vi "SP Add Marker to Plots.vi"(5 "CH Control":T3={"Trace Orientation"=enum."Overlay", "Frequency"={"Change Frequency"=FALSE, "Start"=500.0, "Stop"=1500.0, "Units"=enum."MHz"}, "Markers"=[], "Traces"=[]} {"Traces"."Reference" format="%#.2g"; "Traces"."Display Data" items=["Data", "Memory", "Data/Memory"]; "Traces"."Format" items=["Log Mag", "Phase", "Expanded Phase", "Delay", "Smith", "Polar", "Lin Mag", "SWR", "Loss", "Real", "Imaginary"]; "Traces"."Scale" min=0.001 step=1.0 format="%#.2g"; "Traces"."Position" min=0.0 max=10.0; "Frequency"."Stop" format="%.3g"; "Frequency"."Start" format="%.3g"}, 7 "Plot References":refnum<vi>[](array[refnum]), 8 "error in (no error)":errorcluster, 9 "Marker":T1, 10 "Marker Table":refnum<vi>, 11 "Plot Ref":refnum<vi>) -> (0 "error out":errorcluster)   [LabVIEW 2011]
uses:
  TypeDefs/SP Display Plot Controls Cluster.ctl
  TypeDefs/SP Frequency Units.ctl
  TypeDefs/SP Marker Cluster.ctl
  TypeDefs/SP Marker Type.ctl
  TypeDefs/SP Display Trace Controls.ctl
  TypeDefs/SP Display Format.ctl
  TypeDefs/SP Display Data.ctl
panel:
  # "Div"
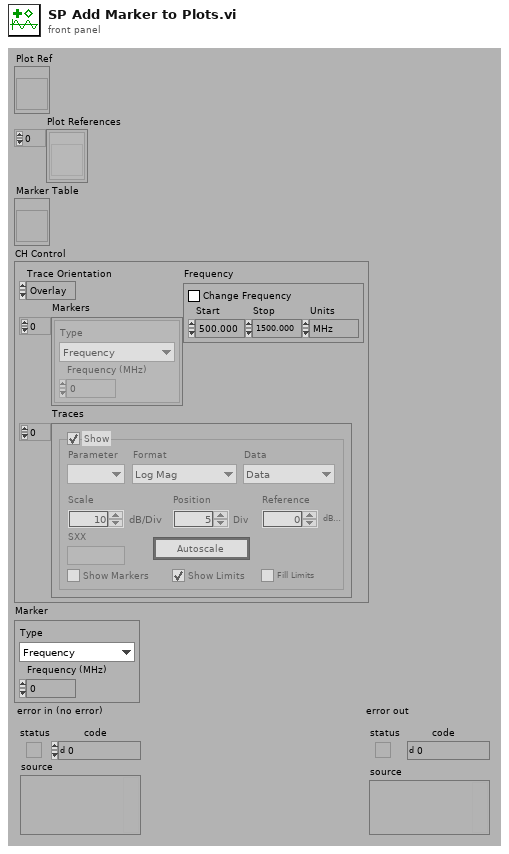
[diagram p1: front panel]
types:
  T1 = typedef "SP Marker Cluster.ctl" = cluster{"Type":T2, "Frequency (MHz)":dbl}
  T2 = typedef "SP Marker Type.ctl" = enum16{"Frequency", "Trace Maximum", "Trace Minimum", "Limit Maximum", "Limit Minimum"}
  T3 = typedef "SP Display Plot Controls Cluster.ctl" = cluster{"Trace Orientation":enum32{"Overlay", "Split"}, "Frequency":cluster{"Change Frequency":bool, "Start":dbl, "Stop":dbl, "Units":T4}, "Markers":T1[], "Traces":T5[]}
  T4 = typedef "SP Frequency Units.ctl" = enum16{"Hz", "kHz", "MHz", "GHz", "Points"}
  T5 = typedef "SP Display Trace Controls.ctl" = cluster{"Trace On":bool, "Measure":i32, "Format":T6, "Autoscale":bool, "Reference":dbl, "\nRefUnit":string, "Position":dbl, "Scale":dbl, "ScaleUnit":string, "LimitOn":bool, "LimitFill":bool, "Display Data":T7, "Show Markers":bool, "SXX":string}
  T6 = typedef "SP Display Format.ctl" = i32
  T7 = typedef "SP Display Data.ctl" = u16
  T8 = typedef "SP Channel Data.ctl" = cluster{"Graph Ref":refnum<vi>, "Data":cluster{"Data":cluster{"X":dbl[], "Y":dbl[]}, "Index":i32}, "ULimits":cluster{"Data":cluster{"X":dbl[], "Y":dbl[]}, "Index":i32}[], "LLimits":cluster{"Data":cluster{"X":dbl[], "Y":dbl[]}, "Index":i32}[]}
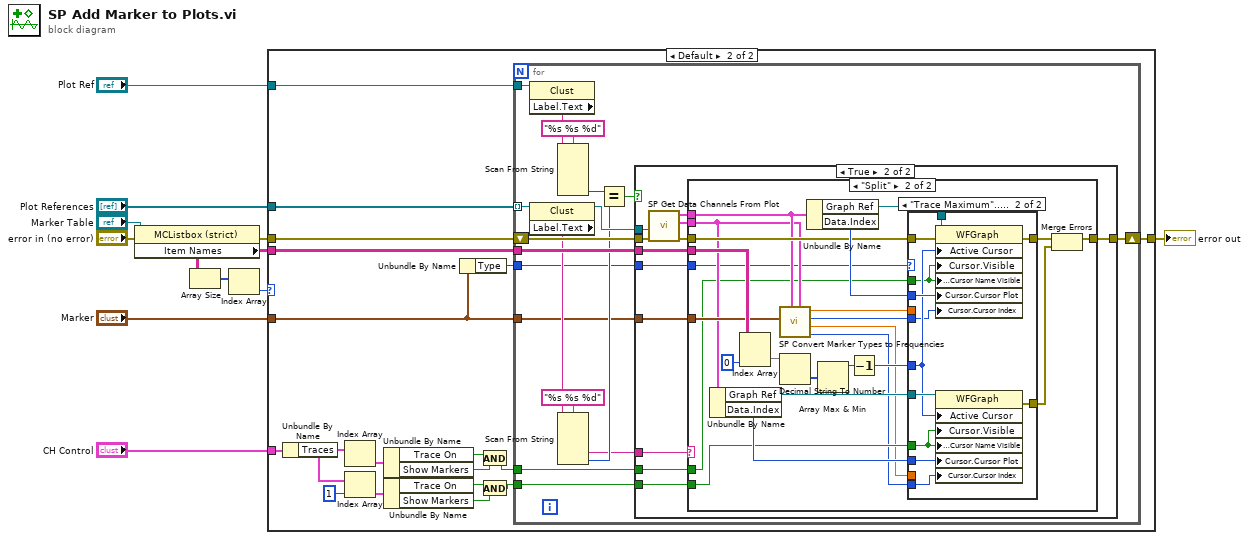
[diagram p0: block diagram]
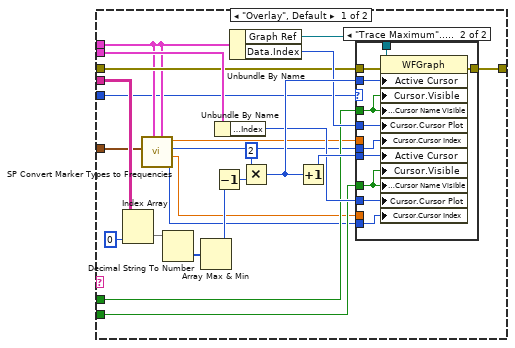
[diagram p4: hidden frame]
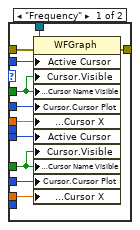
[diagram p5: hidden frame]
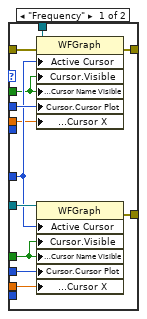
[diagram p6: hidden frame]
diagram:
  n1 = property class="MCListbox (strict)"(reference="Marker Table", error in="error in (no error)") -> (error out=w9:errorcluster, "Item Names"=w6:string[][])  [unwired: 1 out]
  n2 = Array Size(array=w6) -> (size(s)=w7:i32[])
  n3 = Index Array(array=w7) -> (element=w5:i32)  [unwired: 1 in]
  n4 = case shown="Default" w5 {
    tunnel: "Plot References" -> [_ w27]
    tunnel: w9 -> [w12 w30]
    tunnel: [w12 w29] -> w8
    tunnel: w6 -> [_ w28]
    tunnel: "Plot Ref" -> [_ w26]
    tunnel: "Marker" -> [_ w14]
    tunnel: "CH Control" -> [_ w15]
    frame 9.. {
      # "If there are already 8 markers, don't add anymore."
    }
    frame Default {
      n5 = Unbundle By Name(w15) -> ("Traces"=w20:T5[])
      n6 = Index Array(array=w20) -> (element=w21:T5)  [unwired: 1 in]
      n7 = Index Array(array=w20, index=1) -> (element=w22:T5)
      n8 = Unbundle By Name(w21) -> ("Trace On"=w18:bool, "Show Markers"=w19:bool)
      n9 = Unbundle By Name(w22) -> ("Trace On"=w25:bool, "Show Markers"=w24:bool)
      n10 = Unbundle By Name(w14) -> ("Type"=w13:T2)
      n11 = And(x=w18, y=w19) -> (x .and. y?=w17:bool)
      n12 = And(x=w25, y=w24) -> (x .and. y?=w16:bool)
      n13 = for {
        tunnel: w28 -> [w46]
        tunnel: w27 -> [w45] mode=indexing
        tunnel: w26 -> [w41]
        shift-right: [w47] -> w29
        shift-left: w30 -> [w48]
        tunnel: w17 -> [w34]
        tunnel: w16 -> [w33]
        tunnel: w14 -> [w32]
        tunnel: w13 -> [w31]
        n14 = property class="Clust"(reference=w41) -> ("Label.Text"=w39:string)  [unwired: 1 in, 2 out]
        n15 = property class="Clust"(reference=w45) -> (reference out=w44:refnum<vi>, "Label.Text"=w42:string)  [unwired: 1 in, 1 out]
        n16 = Scan From String(format string="%s %s %d", input string=w39) -> (output 3=w38:i32)  [unwired: 2 in, 8 out]
        n17 = Scan From String(format string="%s %s %d", input string=w42) -> (output 2=w35:string, output 3=w37:i32)  [unwired: 2 in, 7 out]
        n18 = Equal?(x=w38, y=w37) -> (x = y?=w36:bool)
        n19 = case shown="True" w36 {
          tunnel: w48 -> [w49 w56]
          tunnel: [w49 w61] -> w47
          tunnel: w46 -> [_ w60]
          tunnel: w44 -> [_ w54]
          tunnel: w35 -> [_ w59]
          tunnel: w34 -> [_ w58]
          tunnel: w33 -> [_ w57]
          tunnel: w32 -> [_ w51]
          tunnel: w31 -> [_ w50]
          frame False {
          }
          frame True {
            n20 = call "SP Get Data Channels From Plot.vi"("error in (no error)"=w56, "Plot Ref"=w54) -> ("error out"=w55:errorcluster, "CH 2"=w53:T8, "CH 1"=w52:T8)  [unwired: 7 out]
            n21 = case shown="\"Split\"" w59 {
              tunnel: w55 -> [w69 w117]
              tunnel: [w85 w127] -> w61
              tunnel: w60 -> [w80 w128]
              tunnel: w58 -> [w72 w113]
              tunnel: w57 -> [w71 w118]
              tunnel: w53 -> [w70 w114]
              tunnel: w52 -> [w68 w115]
              tunnel: w51 -> [w67 w116]
              tunnel: w50 -> [w66 w112]
              frame "Overlay", Default {
                n22 = Index Array(array=w80, index (col)=0 ("disabled index (col)")) -> (element=w83:string[])  [unwired: 1 in]
                n23 = call "SP Convert Marker Types to Frequencies.vi"("CH 2"=w68, "CH 1"=w68, "Marker"=w67) -> ("CH2 Index"=w63:i32, "CH2 Frequency"=w64:dbl, "CH1 Index"=w62:i32, "CH1 Frequency"=w65:dbl)  [unwired: 3 out]
                n24 = Decimal String To Number(string=w83) -> (number=w82:i32[])  [unwired: 3 out]
                n25 = Array Max & Min(array=w82) -> (max value=w74:i32)  [unwired: 3 out]
                n26 = Decrement(x=w74) -> (x-1=w73:i32)
                n27 = Unbundle By Name(w70) -> ("Data.Index"=w75:i32)
                n28 = Unbundle By Name(w68) -> ("Graph Ref"=w76:refnum<vi>, "Data.Index"=w77:i32)
                n29 = Multiply(x=2 ("y"), y=w73) -> (x*y=w78:i32)
                n30 = Increment(x=w78) -> (x+1=w79:i32)
                n31 = case shown="\"Trace Maximum\"..\"Limit Minimum\"" w66 {
                  tunnel: [w96 w107] -> w85
                  tunnel: w79 -> [w95 w106]
                  tunnel: w78 -> [w94 w105]
                  tunnel: w77 -> [w93 w104]
                  tunnel: w76 -> [w92 w103]
                  tunnel: w75 -> [w91 w102]
                  tunnel: w72 -> [w90 w101]
                  tunnel: w71 -> [w89 w100]
                  tunnel: w69 -> [w88 w99]
                  tunnel: w65 -> [w87 _]
                  tunnel: w64 -> [w86 _]
                  tunnel: w63 -> [_ w98]
                  tunnel: w62 -> [_ w97]
                  frame "Frequency" {
                    n32 = property class="WFGraph"(reference=w92, error in=w88, "Active Cursor"=w94, "Cursor.Visible"=w90, "Cursor.Cursor Name Visible"=w90, "Cursor.Cursor Plot"=w93, "Cursor.Cursor Position:Cursor X"=w87, "Active Cursor"=w95, "Cursor.Visible"=w89, "Cursor.Cursor Name Visible"=w89, "Cursor.Cursor Plot"=w91, "Cursor.Cursor Position:Cursor X"=w86) -> (error out=w96:errorcluster)  [unwired: 1 out]
                  }
                  frame "Trace Maximum".."Limit Minimum" {
                    n33 = property class="WFGraph"(reference=w103, error in=w99, "Active Cursor"=w105, "Cursor.Visible"=w101, "Cursor.Cursor Name Visible"=w101, "Cursor.Cursor Plot"=w104, "Cursor.Cursor Index"=w97, "Active Cursor"=w106, "Cursor.Visible"=w100, "Cursor.Cursor Name Visible"=w100, "Cursor.Cursor Plot"=w102, "Cursor.Cursor Index"=w98) -> (error out=w107:errorcluster)  [unwired: 1 out]
                  }
                }
              }
              frame "Split" {
                n34 = Unbundle By Name(w114) -> ("Graph Ref"=w122:refnum<vi>, "Data.Index"=w121:i32)
                n35 = Index Array(array=w128, index (col)=0 ("disabled index (col)")) -> (element=w130:string[])  [unwired: 1 in]
                n36 = call "SP Convert Marker Types to Frequencies.vi"("CH 2"=w114, "CH 1"=w115, "Marker"=w116) -> ("CH2 Index"=w109:i32, "CH2 Frequency"=w110:dbl, "CH1 Index"=w108:i32, "CH1 Frequency"=w111:dbl)  [unwired: 3 out]
                n37 = Decimal String To Number(string=w130) -> (number=w129:i32[])  [unwired: 3 out]
                n38 = Unbundle By Name(w115) -> ("Graph Ref"=w123:refnum<vi>, "Data.Index"=w124:i32)
                n39 = Array Max & Min(array=w129) -> (max value=w120:i32)  [unwired: 3 out]
                n40 = Decrement(x=w120) -> (x-1=w119:i32)
                n41 = case shown="\"Trace Maximum\"..\"Limit Minimum\"" w112 {
                  tunnel: [w143 w155] -> w126
                  tunnel: [w142 w154] -> w125
                  tunnel: w124 -> [w141 w153]
                  tunnel: w123 -> [w140 w152]
                  tunnel: w122 -> [w139 w151]
                  tunnel: w121 -> [w138 w150]
                  tunnel: w119 -> [w137 w149]
                  tunnel: w118 -> [w136 w148]
                  tunnel: w117 -> [w135 w147]
                  tunnel: w113 -> [w134 w146]
                  tunnel: w111 -> [w133 _]
                  tunnel: w110 -> [w132 _]
                  tunnel: w109 -> [_ w144]
                  tunnel: w108 -> [_ w145]
                  frame "Frequency" {
                    n42 = property class="WFGraph"(reference=w140, error in=w135, "Active Cursor"=w137, "Cursor.Visible"=w134, "Cursor.Cursor Name Visible"=w134, "Cursor.Cursor Plot"=w141, "Cursor.Cursor Position:Cursor X"=w133) -> (error out=w143:errorcluster)  [unwired: 1 out]
                    n43 = property class="WFGraph"(reference=w139, "Active Cursor"=w137, "Cursor.Visible"=w136, "Cursor.Cursor Name Visible"=w136, "Cursor.Cursor Plot"=w138, "Cursor.Cursor Position:Cursor X"=w132) -> (error out=w142:errorcluster)  [unwired: 1 in, 1 out]
                  }
                  frame "Trace Maximum".."Limit Minimum" {
                    n44 = property class="WFGraph"(reference=w152, error in=w147, "Active Cursor"=w149, "Cursor.Visible"=w146, "Cursor.Cursor Name Visible"=w146, "Cursor.Cursor Plot"=w153, "Cursor.Cursor Index"=w145) -> (error out=w155:errorcluster)  [unwired: 1 out]
                    n45 = property class="WFGraph"(reference=w151, "Active Cursor"=w149, "Cursor.Visible"=w148, "Cursor.Cursor Name Visible"=w148, "Cursor.Cursor Plot"=w150, "Cursor.Cursor Index"=w144) -> (error out=w154:errorcluster)  [unwired: 1 in, 1 out]
                  }
                }
                n46 = Merge Errors(w126, w125) -> (w127:errorcluster)
              }
            }
          }
        }
      }
    }
  }
  "error out" <- w8
